vi "Filter Indicator Terms.vi"(11 "Terms[]":refnum<vi>[](array[refnum])) -> (3 "Terms[] out":refnum<vi>[](array[refnum]))   [LabVIEW 2020, in "CSM-Helper.lvclass"]
uses:
  CSM-Helper.lvclass
  CSM-Helper.lvclass/CSM-Helper.ctl
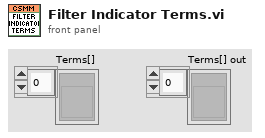
[diagram p1: front panel]
types:
  T1 = typedef "LVPositionTypeDef.ctl" = cluster{"Left":i32, "Top":i32}
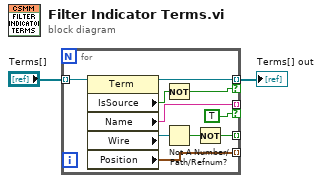
[diagram p0: block diagram]
diagram:
  n1 = for {
    tunnel: "Terms[]" -> [w12] mode=indexing
    tunnel: [w11] -> _ mode=indexing if=TRUE
    tunnel: [w8] -> _ mode=indexing
    tunnel: [w6] -> _ mode=indexing
    tunnel: [w5] -> w1 mode=indexing if=w4
    n2 = property class="Term"(reference=w12) -> (reference out=w5:refnum<vi>, "IsSource"=w10:bool, "Name"=w11:string, "Wire"=w9:refnum<vi>, "Position"=w6:T1)  [unwired: 1 in, 1 out]
    n3 = Not(x=w10) -> (.not. x?=w4:bool)
    n4 = Not A Number/Path/Refnum?(number/path/refnum=w9) -> (NaN/Path/Refnum?=w3:bool)
    n5 = Not(x=w3) -> (.not. x?=w8:bool)
  }
  "Terms[] out" <- w1
